vi "User Authentication.vi"(8 "error in":errorcluster, 11 "file path":path=path "E:/Temporary Code Modification/User Interface Testbench v2.0/User interface plan.xlsx") -> (0 "error out":errorcluster, 1 "USER EXISTS?":bool, 2 "user?":string, 3 "Exit button pressed":bool, 5 "Authentication message":string)   [LabVIEW 2019, in "ZenGage v3.0 UI.lvclass"]
uses:
  ZenGage v3.0 UI.lvclass
  Common/Controls/Pop-up Input.ctl
panel:
  in  "Exit":bool
  out "Proceed? 2":bool
  in  "Ok button":bool
  in  "PASSWORD":string
  in  "USER ID":string
  out "Popup Title":string="     USER AUTHENTICATION"
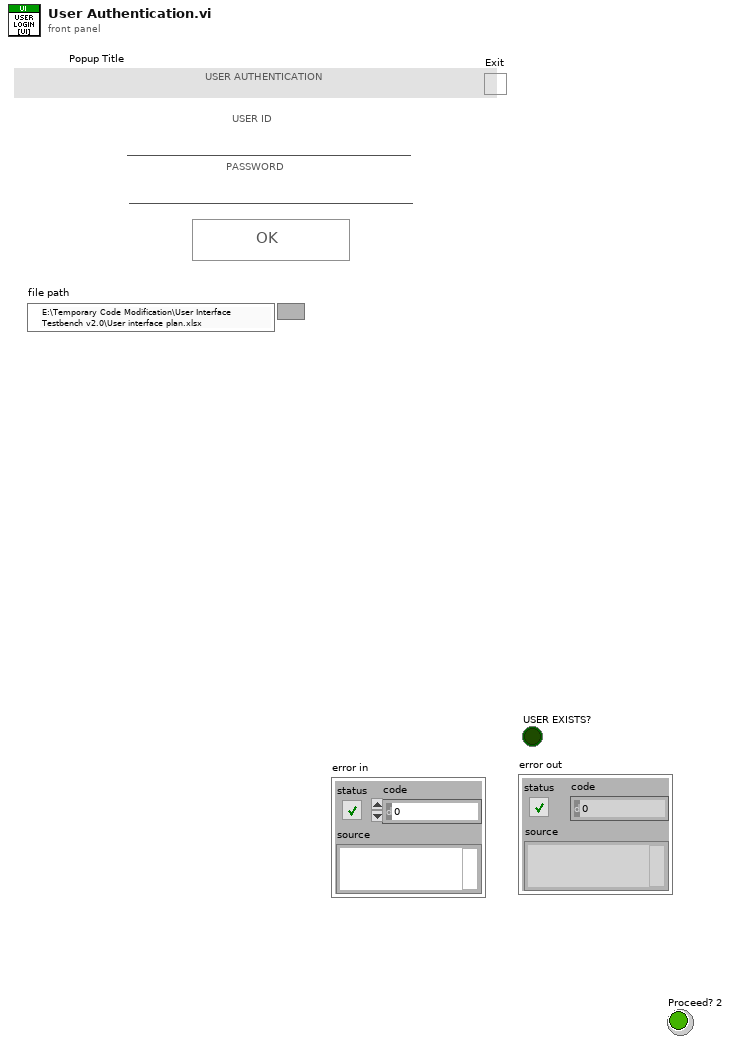
[diagram p1: front panel]
types:
  T1 = enum32{"Invalid", "Standard", "Closed", "Hidden", "Minimized", "Maximized"}
  T2 = enum8{"Enabled", "Disabled", "Disabled and Grayed Out"}
  T3 = typedef "Pop-up Input.ctl" = cluster{"Pop-up Type":enum16{"Open Logo Display", "Close Logo Display", "Open Loading Bar", "Close Loading Bar", "Open Alert Display", "Close Alert Display", "One button dialog box", "Two button dialog box", "User Authentication"}, "Title":string, "Message":string, "Button 1 Text":string, "Button 2 Text":string, "Show Close? T/F":bool, "Title Blink? T/F":bool, "Title Blink Colour":u32}
  T4 = typedef "ZenGage v3.0 UI.lvclass/Pop-up Output.ctl" = cluster{"Pop-up Type":enum16{"Open Logo Display", "Close Logo Display", "Open Loading Bar", "Close Loading Bar", "Open Alert Display", "Close Alert Display", "One button dialog box", "Two button dialog box", "User Authentication"}, "Message":string, "Pressed Button":string}
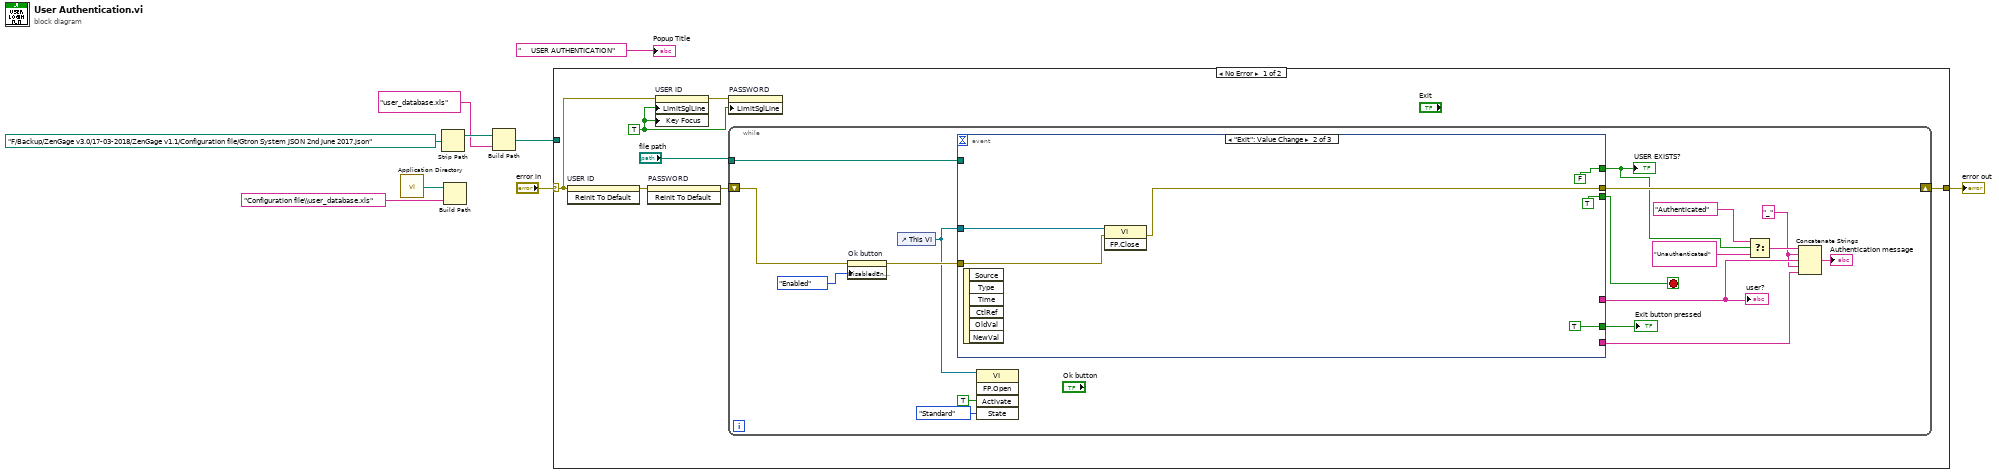
[diagram p0: block diagram]
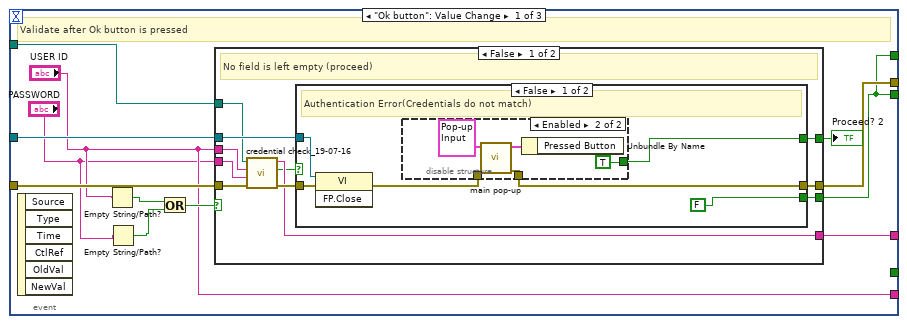
[diagram p2: hidden frame]
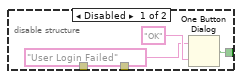
[diagram p3: hidden frame]
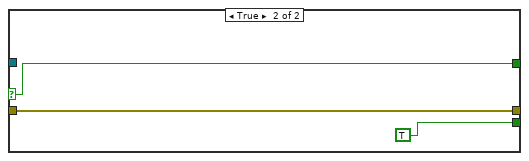
[diagram p4: hidden frame]
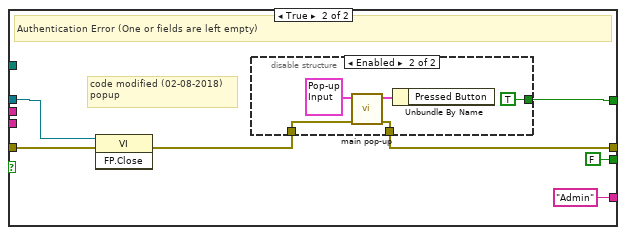
[diagram p5: hidden frame]
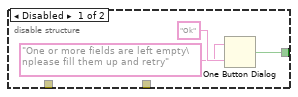
[diagram p6: hidden frame]
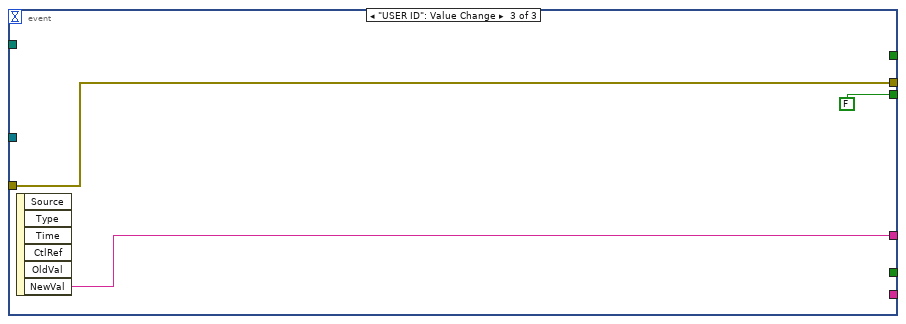
[diagram p7: hidden frame]
diagram:
  n1 = call <vilib>:"Application Directory.vi"() -> ("Application Directory"=w2:path)
  n2 = Strip Path(path=path "F:/Backup/ZenGage v3.0/17-03-2018/ZenGage v1.1/Configuration file/Gtron System JSON 2nd June 2017.json") -> (stripped path=w6:path)  [unwired: 1 out]
  n3 = Build Path(base path=w2, name or relative path="Configuration file\\user_database.xls") -> ()  [unwired: 1 out]
  n4 = Build Path(base path=w6, name or relative path="user_database.xls") -> (appended path=w5:path)
  n5 = case shown="No Error" "error in" {
    selector: "error in" -> [w12 w98]
    tunnel: [w16 w98] -> w8
    tunnel: w5 -> [_ _]
    frame No Error {
      w11 = TRUE
      n6 = invoke on="USER ID" class="Str" method="Reinit To Default"(error in=w12) -> (error out=w15:errorcluster)  [unwired: 2 in, 2 out]
      n7 = invoke on="PASSWORD" class="Str" method="Reinit To Default"(error in=w15) -> (error out=w14:errorcluster)  [unwired: 2 in, 2 out]
      n8 = property on="USER ID" class="Str"(error in=w12, "LimitSglLine"=w11, "Key Focus"=w11) -> (error out=w13:errorcluster)  [unwired: 1 in, 1 out]
      n9 = property on="PASSWORD" class="Str"(error in=w13, "LimitSglLine"=w11) -> ()  [unwired: 1 in, 2 out]
      n10 = while {
        shift-right: [w30] -> w16
        shift-left: w14 -> [w33]
        tunnel: "file path" -> [w28]
        stop <- w26 stop-if-true
        w20 = "_" ("string")
        n11 = property on="Ok button" class="Bool"(error in=w33, "DisabledEnum"=T2."Enabled" ("Disabled")) -> (error out=w31:errorcluster)  [unwired: 1 in, 1 out]
        n12 = control-ref of="This VI"() -> (w29:refnum<vi>)
        n13 = event shown="[1] \"Exit\": Value Change" {
          selector: _ -> [_ _ _]
          dyn-events: _ -> [_ _ _]
          timeout: _ -> [_ _ _]
          tunnel: w31 -> [w46 w93 w97]
          tunnel: [w45 w92 w97] -> w30
          tunnel: w29 -> [w44 w94 _]
          tunnel: [w39 TRUE ("USER EXISTS?") FALSE ("USER EXISTS?")] -> w26
          tunnel: [w43 _ w95] -> w21
          tunnel: w28 -> [w40 _ _]
          tunnel: [w39 FALSE _] -> w23
          tunnel: ["USER ID" _ _] -> w19
          tunnel: [_ TRUE _] -> w17
          event "Ok button": Value Change {
            # "Validate after Ok button is pressed"
            n14 = event-data() -> ()  [unwired: 1 in, 6 out]
            n15 = Empty String/Path?(string/path="USER ID") -> (empty?=w37:bool)
            n16 = Empty String/Path?(string/path="PASSWORD") -> (empty?=w35:bool)
            n17 = Or(x=w37, y=w35) -> (x .or. y?=w42:bool)
            n18 = case shown="False" w42 {
              tunnel: w46 -> [w47 w78]
              tunnel: [w56 w74] -> w45
              tunnel: w44 -> [w55 w77]
              tunnel: "USER ID" -> [w54 _]
              tunnel: "PASSWORD" -> [w53 _]
              tunnel: [w52 "Admin" ("user?")] -> w43
              tunnel: [w49 FALSE ("USER EXISTS?")] -> w39
              tunnel: [w50 w76] -> w41
              tunnel: w40 -> [w48 _]
              frame False {
                # "No field is left empty (proceed)"
                n19 = call "credential check_19-07-16.vi"("error in"=w47, "PASSWORD"=w53, "USER NAME"=w54, "file path (dialog if empty)"=w48) -> ("error out"=w57:errorcluster, "USER EXISTS?"=w51:bool, "user?"=w52:string)  [unwired: 5 in]
                n20 = case shown="False" w51 {
                  selector: w51 -> [_ w72]
                  tunnel: w57 -> [w63 w73]
                  tunnel: [w58 w73] -> w56
                  tunnel: w55 -> [w62 _]
                  tunnel: [w60 w72] -> w50
                  tunnel: [FALSE TRUE] -> w49
                  frame False {
                    # "Authentication Error(Credentials do not match)"
                    n21 = invoke class="VI" method="FP.Close"(reference=w62, error in=w63) -> (error out=w59:errorcluster)  [unwired: 1 in, 2 out]
                    n22 = disable-structure shown="Enabled" {
                      disable-tunnel: [w66 TRUE ("true")] -> w60
                      disable-tunnel: w59 -> [_ _]
                      disable-tunnel: [_ w68] -> w58
                      frame Disabled {
                        n23 = One Button Dialog(message="User Login Failed", button name ("OK")="OK" ("Boolean Text.Text")) -> (true=w66:bool)
                      }
                      frame Enabled {
                        n24 = call "main pop-up.vi"("Pop-up Input"=T3 {"Pop-up Type"=enum."One button dialog box", "Title"="ALERT", "Message"="User login failed", "Button 1 Text"="OK", "Button 2 Text"="", "Show Close? T/F"=FALSE, "Title Blink? T/F"=FALSE, "Title Blink Colour"=0}) -> ("error out"=w68:errorcluster, "Pop-up Output"=w70:T4)  [unwired: 9 in]
                        n25 = Unbundle By Name(w70) -> ()  [unwired: 1 out]
                      }
                    }
                  }
                  frame True {
                  }
                }
              }
              frame True {
                # "code modified (02-08-2018)\npopup"
                # "Authentication Error (One or fields are left empty)"
                n26 = invoke class="VI" method="FP.Close"(reference=w77, error in=w78) -> (error out=w75:errorcluster)  [unwired: 1 in, 2 out]
                n27 = disable-structure shown="Enabled" {
                  disable-tunnel: [w81 TRUE ("true")] -> w76
                  disable-tunnel: w75 -> [_ w86]
                  disable-tunnel: [_ w85] -> w74
                  frame Disabled {
                    n28 = One Button Dialog(message="One or more fields are left empty\nplease fill them up and retry" ("Message Input"), button name ("OK")="Ok" ("Boolean Text.Text")) -> (true=w81:bool)
                  }
                  frame Enabled {
                    n29 = call "main pop-up.vi"("error in"=w86, "Pop-up Input"=T3 {"Pop-up Type"=enum."One button dialog box", "Title"="ALERT", "Message"="One or more fields are left empty\nplease fill them up and retry", "Button 1 Text"="OK", "Button 2 Text"="", "Show Close? T/F"=FALSE, "Title Blink? T/F"=FALSE, "Title Blink Colour"=0}) -> ("error out"=w85:errorcluster, "Pop-up Output"=w88:T4)  [unwired: 8 in]
                    n30 = Unbundle By Name(w88) -> ()  [unwired: 1 out]
                  }
                }
              }
            }
            "Proceed? 2" <- w41
          }
          event "Exit": Value Change {
            n31 = event-data() -> ()  [unwired: 1 in, 6 out]
            n32 = invoke class="VI" method="FP.Close"(reference=w94, error in=w93) -> (error out=w92:errorcluster)  [unwired: 1 in, 2 out]
          }
          event "USER ID": Value Change {
            n33 = event-data() -> ("NewVal"=w95:string)  [unwired: 1 in, 5 out]
          }
        }
        "USER EXISTS?" <- w23
        "user?" <- w21
        "Exit button pressed" <- w17
        n34 = invoke class="VI" method="FP.Open"(reference=w29, "Activate"=TRUE ("Activate?"), "State"=T1."Standard") -> ()  [unwired: 2 in, 5 out]
        n35 = Select(t="Authenticated", s=w23, f="Unauthenticated") -> (s? t:f=w22:string)
        n36 = Concatenate Strings(w22, w20, w21, w20, w19) -> (→"Authentication message":string)
      }
    }
    frame Error {
    }
  }
  "error out" <- w8
  "Popup Title" <- "     USER AUTHENTICATION" ("Dialog Box out")
